vi "Result Type.vi"(11 "Future in":refnum<class "Future.lvclass">) -> (2 "Result Type":refnum<class "Value.lvclass">)   [LabVIEW 2020, in "Promises.lvlib" / "Future.lvclass"]
uses:
  Future.lvclass
  Value/Value.lvclass
  Future.lvclass/Future.ctl
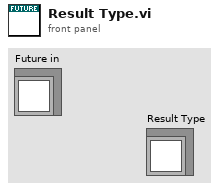
[diagram p1: front panel]
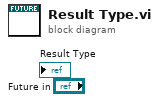
[diagram p0: block diagram]
diagram:
